vi "ReceiveTcpMessageBase.vi"(6 "timeout (5 sec)":i32=5000, 8 "error in (no error)":errorcluster, 11 "tcp in":refnum<k5>) -> (0 "error out":errorcluster, 1 "timed out":bool, 2 "Message":T1, 3 "tcp out":refnum<k5>, 4 "bytes received":i32, 5 "ByteReadErrors":bool[](array[boolean]))   [LabVIEW 2017]
uses:
  <vilib>/addons/InsightCM/MessageBus/Base/controls/Message.ctl
  <vilib>/addons/InsightCM/MessageBus/Base/controls/MessageHeader.ctl
  <vilib>/addons/InsightCM/MessageBus/Base/controls/KeyValuePair.ctl
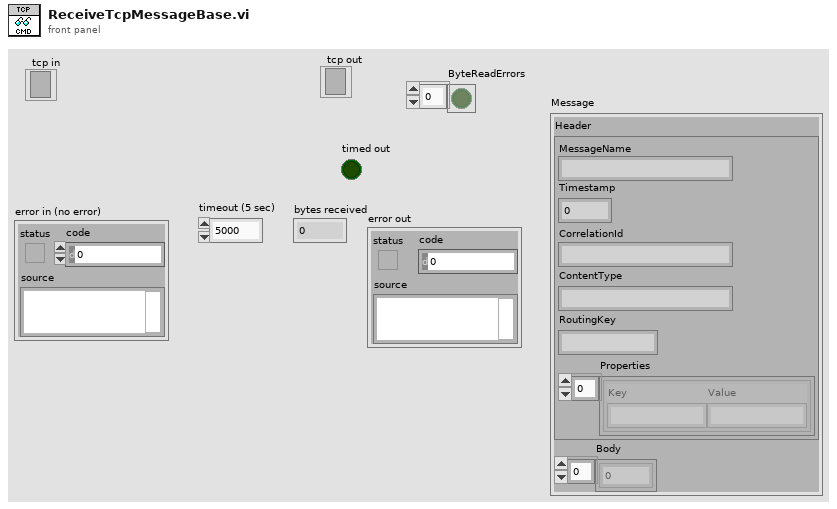
[diagram p1: front panel]
types:
  T1 = typedef "Message.ctl" = cluster{"Header":T2, "Body":u8[]}
  T2 = typedef "MessageHeader.ctl" = cluster{"MessageName":string, "Timestamp":i64, "CorrelationId":string, "ContentType":string, "RoutingKey":string, "Properties":T3[]}
  T3 = typedef "KeyValuePair.ctl" = cluster{"Key":string, "Value":string}
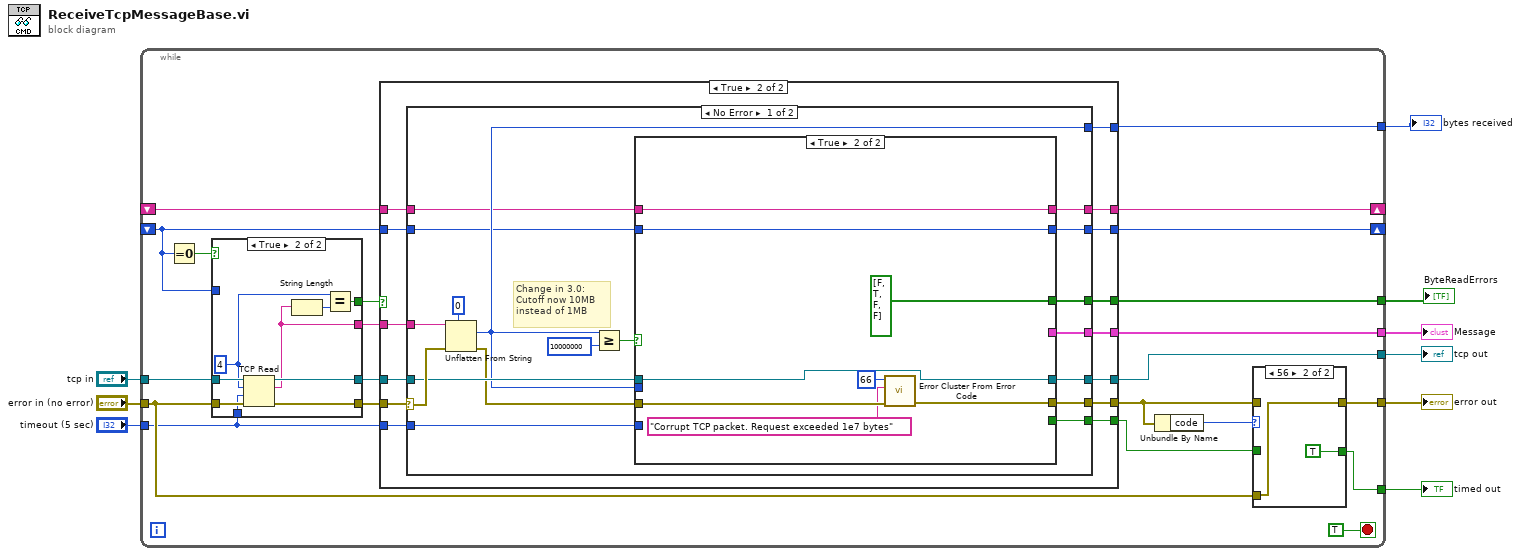
[diagram p0: block diagram]
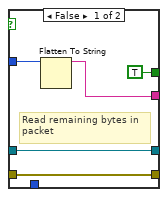
[diagram p2: hidden frame]
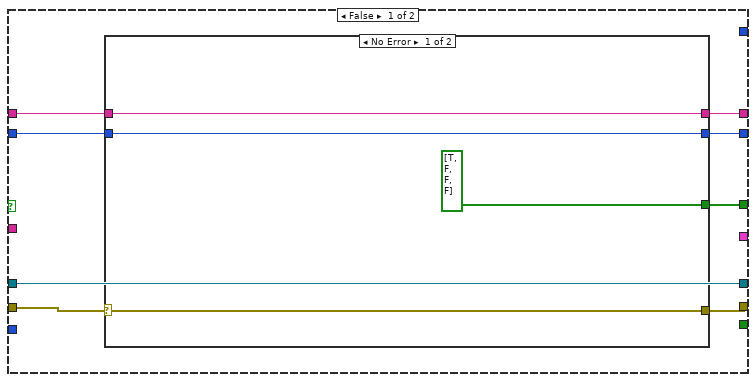
[diagram p3: hidden frame]
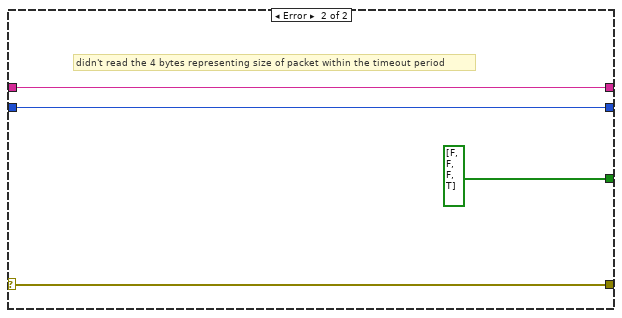
[diagram p4: hidden frame]
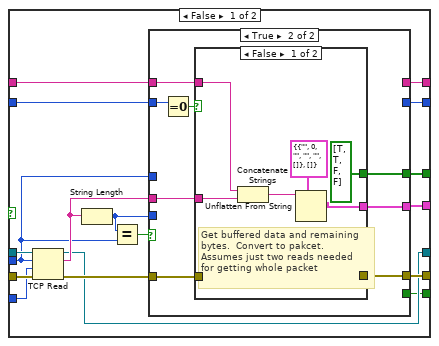
[diagram p5: hidden frame]
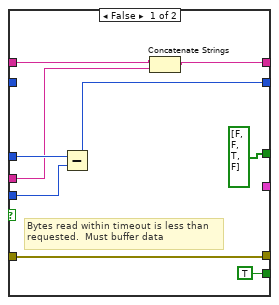
[diagram p6: hidden frame]
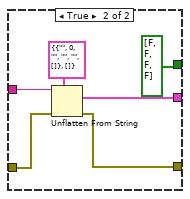
[diagram p7: hidden frame]
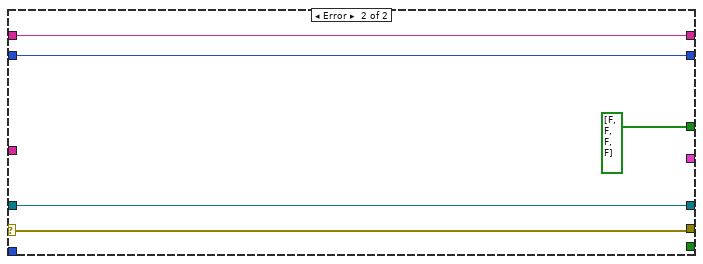
[diagram p8: hidden frame]
diagram:
  n1 = while {
    tunnel: "timeout (5 sec)" -> [w10]
    tunnel: [w29] -> w8
    tunnel: [w28] -> w7
    tunnel: "tcp in" -> [w27]
    tunnel: [w26] -> w5
    tunnel: [w24] -> w4
    tunnel: "error in (no error)" -> [w22]
    tunnel: [w21] -> w2
    tunnel: [w18] -> w1
    shift-right: [w16] -> _
    shift-left: _ -> [w14]
    shift-right: [w15] -> _
    shift-left: _ -> [w11]
    stop <- TRUE stop-if-true
    n2 = Equal To 0?(x=w11) -> (x = 0?=w12:bool)
    n3 = case shown="True" w12 {
      tunnel: [w32 w45] -> w31
      tunnel: [w33 w44] -> w30
      tunnel: w27 -> [w33 w43]
      tunnel: w22 -> [w32 w42]
      tunnel: [w34 w41] -> w20
      tunnel: [TRUE w38] -> w19
      tunnel: w11 -> [w35 _]
      tunnel: w10 -> [_ w37]
      frame False {
        # "Read remaining bytes in\npacket"
        n4 = Flatten To String(anything=w35) -> (data string=w34:string)  [unwired: 3 in, 2 out]
      }
      frame True {
        w40 = 4 ("bytes to read")
        n5 = TCP Read(connection ID=w43, bytes to read=w40, error in (no error)=w42, 9:w37) -> (connection ID out=w44:refnum<k5>, data out=w41:string, error out=w45:errorcluster)  [unwired: 1 in]
        n6 = String Length(string=w41) -> (length=w39:i32)
        n7 = Equal?(x=w40, y=w39) -> (x = y?=w38:bool)
      }
    }
    n8 = case shown="True" w19 {
      tunnel: w31 -> [w51 w75]
      tunnel: w30 -> [w53 w74]
      tunnel: w10 -> [_ w73]
      tunnel: [_ w72] -> w29
      tunnel: [_ w71] -> w28
      tunnel: [w53 w70] -> w26
      tunnel: [w50 w69] -> w23
      tunnel: [w52 w68] -> w18
      tunnel: w20 -> [_ w67]
      tunnel: [w48 w66] -> w16
      tunnel: [w46 w65] -> w15
      tunnel: w14 -> [w49 w64]
      tunnel: w11 -> [w47 w63]
      tunnel: [_ w62] -> w13
      frame False {
        n9 = case shown="No Error" w51 {
          selector: w51 -> [w56 w61]
          tunnel: [bool[] [TRUE, FALSE, FALSE, FALSE] bool[] [FALSE, FALSE, FALSE, TRUE]] -> w52
          tunnel: [w56 w61] -> w50
          tunnel: w49 -> [w55 w59]
          tunnel: [w55 w59] -> w48
          tunnel: w47 -> [w54 w58]
          tunnel: [w54 w58] -> w46
          frame No Error {
          }
          frame Error {
            # "didn't read the 4 bytes representing size of packet within the timeout period"
          }
        }
      }
      frame True {
        n10 = case shown="No Error" w75 {
          selector: w75 -> [w91 w152]
          tunnel: w74 -> [w90 w153]
          tunnel: w67 -> [w92 _]
          tunnel: w73 -> [w87 _]
          tunnel: [w88 _] -> w71
          tunnel: [w86 w153] -> w70
          tunnel: [w85 w152] -> w69
          tunnel: [w81 _] -> w72
          tunnel: [w82 bool[] [FALSE, FALSE, FALSE, FALSE]] -> w68
          tunnel: [w80 w149] -> w66
          tunnel: [w79 w150] -> w65
          tunnel: w64 -> [w78 w149]
          tunnel: w63 -> [w77 w150]
          tunnel: [w76 _] -> w62
          frame No Error {
            # "Change in 3.0:\nCutoff now 10MB\ninstead of 1MB"
            n11 = Unflatten From String(type=0 ("length"), binary string=w92, error in (no error)=w91) -> (value=w81:i32, error out=w89:errorcluster)  [unwired: 2 in, 1 out]
            n12 = Greater Or Equal?(x=w81, y=10000000) -> (x >= y?=w83:bool)
            n13 = case shown="True" w83 {
              tunnel: w90 -> [w110 w148]
              tunnel: w89 -> [w109 w147]
              tunnel: [w107 _] -> w88
              tunnel: w87 -> [w106 _]
              tunnel: [w100 w148] -> w86
              tunnel: [w105 w146] -> w85
              tunnel: w81 -> [w98 _]
              tunnel: [w103 bool[] [FALSE, TRUE, FALSE, FALSE]] -> w82
              tunnel: [w99 w142] -> w80
              tunnel: [w97 w141] -> w79
              tunnel: w78 -> [w95 w142]
              tunnel: w77 -> [w94 w141]
              tunnel: [w96 _] -> w76
              frame False {
                n14 = TCP Read(connection ID=w110, bytes to read=w98, error in (no error)=w109, 9:w106) -> (connection ID out=w100:refnum<k5>, data out=w102:string, error out=w108:errorcluster)  [unwired: 1 out]
                n15 = String Length(string=w102) -> (length=w101:i32)
                n16 = Equal?(x=w101, y=w98) -> (x = y?=w104:bool)
                n17 = case shown="True" w104 {
                  tunnel: w108 -> [w119 w127]
                  tunnel: [_ w126] -> w107
                  tunnel: [w119 w125] -> w105
                  tunnel: w102 -> [w112 w124]
                  tunnel: [bool[] [FALSE, FALSE, TRUE, FALSE] w120] -> w103
                  tunnel: w101 -> [w116 _]
                  tunnel: [w111 _] -> w99
                  tunnel: w98 -> [w117 _]
                  tunnel: [w115 _] -> w97
                  tunnel: [TRUE _] -> w96
                  tunnel: w95 -> [w113 w121]
                  tunnel: w94 -> [_ w123]
                  frame False {
                    # "Bytes read within timeout is less than\nrequested.  Must buffer data"
                    n18 = Subtract(x=w117, y=w116) -> (x-y=w115:i32)
                    n19 = Concatenate Strings(w113, w112) -> (w111:string)
                  }
                  frame True {
                    n20 = Equal To 0?(x=w123) -> (x = 0?=w122:bool)
                    n21 = case shown="False" w122 {
                      tunnel: w127 -> [w129 w140]
                      tunnel: [w131 w139] -> w126
                      tunnel: [w129 w138] -> w125
                      tunnel: w124 -> [w133 w137]
                      tunnel: w121 -> [w134 _]
                      tunnel: [bool[] [TRUE, TRUE, FALSE, FALSE] bool[] [FALSE, FALSE, FALSE, FALSE]] -> w120
                      frame False {
                        # "Get buffered data and remaining\nbytes.  Convert to pakcet.\nAssumes just two reads needed\nfor getting whole packet"
                        n22 = Concatenate Strings(w134, w133) -> (w130:string)
                        n23 = Unflatten From String(type=T1 {"Header"={"MessageName"="", "Timestamp"=0, "CorrelationId"="", "ContentType"="", "RoutingKey"="", "Properties"=[]}, "Body"=[]} ("Message"), binary string=w130) -> (value=w131:T1)  [unwired: 3 in, 2 out]
                      }
                      frame True {
                        n24 = Unflatten From String(type=T1 {"Header"={"MessageName"="", "Timestamp"=0, "CorrelationId"="", "ContentType"="", "RoutingKey"="", "Properties"=[]}, "Body"=[]} ("Message"), binary string=w137, error in (no error)=w140) -> (value=w139:T1, error out=w138:errorcluster)  [unwired: 2 in, 1 out]
                      }
                    }
                  }
                }
              }
              frame True {
                n25 = call <vilib>:"Error Cluster From Error Code.vi"("error in (no error)"=w147, "error message (\"\")"="Corrupt TCP packet. Request exceeded 1e7 bytes" ("error message (\"\")"), "error code (0)"=66) -> ("error out"=w146:errorcluster)  [unwired: 6 in]
              }
            }
          }
          frame Error {
          }
        }
      }
    }
    n26 = Unbundle By Name(w23) -> ("code"=w25:i32)
    n27 = case shown="56" w25 {
      tunnel: [w155 w157] -> w24
      tunnel: w23 -> [w155 _]
      tunnel: w22 -> [_ w157]
      tunnel: [w154 TRUE] -> w21
      tunnel: w13 -> [w154 _]
      frame Default {
      }
      frame 56 {
      }
    }
  }
  "error out" <- w4
  "bytes received" <- w8
  "Message" <- w7
  "tcp out" <- w5
  "timed out" <- w2
  "ByteReadErrors" <- w1
